vi "timming_array_to_digital_waveform.vi"(3 "timing array":dbl[](array[numeric])) -> (0 "digital waveform":digitalwaveform(waveform)={"t0"=timestamp(0 s since 1904-01-01), "dt"=0.0, "Y"={"transitions"=[], "data"=[]}, "error"={"status"=FALSE, "code"=37421928, "source"=""}})   [LabVIEW 2011]
doc: "takes the timing info recieved from the DG645 Delay generator and transforms it into a digital waveform graph.\nMakes sure, all timings are setup in reference to t0!"
uses:
  <vilib>/Waveform/DWDTOps.llb/DWDT Boolean Array to Digital.vi
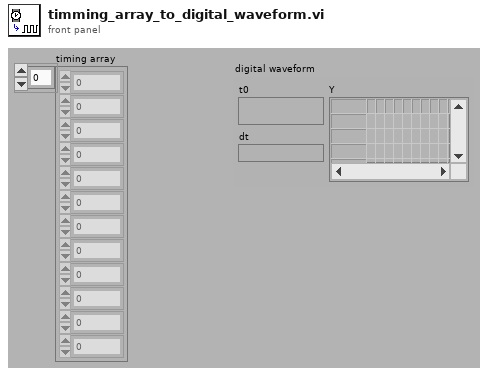
[diagram p1: front panel]
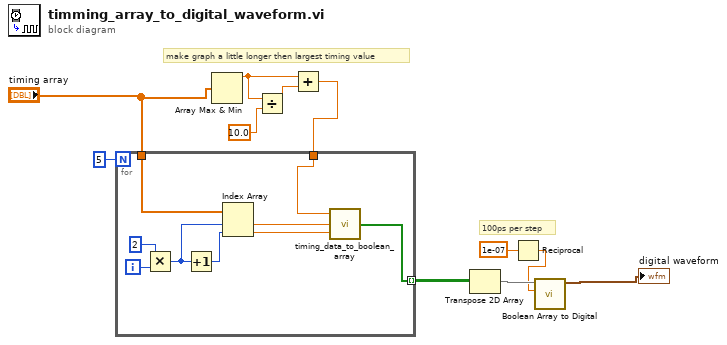
[diagram p0: block diagram]
diagram:
  # "100ps per step"
  # "make graph a little longer then largest timing value"
  n1 = Array Max & Min(array="timing array") -> (max value=w5:dbl)  [unwired: 3 out]
  n2 = Divide(x=w5, y=10.0) -> (x/y=w4:dbl)
  n3 = Add(x=w5, y=w4) -> (x+y=w3:dbl)
  n4 = for {
    N: 5 -> [_]
    tunnel: [w18] -> w10 mode=indexing
    tunnel: w3 -> [w17]
    tunnel: "timing array" -> [w16]
    i -> [w20]
    n5 = Multiply(x=2, y=w20) -> (x*y=w12:i32)
    n6 = Increment(x=w12) -> (x+1=w15:i32)
    n7 = Index Array(array=w16, index #1=w12, index #2=w15) -> (element #1=w14:dbl, element #2=w13:dbl)
    n8 = call "timing_data_to_boolean_array.vi"("end time [us]"=w13, "start time [us]"=w14, "overall length [us]"=w17) -> ("boolean timing array"=w18:bool[])  [unwired: 1 in]
  }
  n9 = Transpose 2D Array(2D array=w10) -> (transposed array=w9:bool[][])
  n10 = Reciprocal(x=1e-07) -> (1/x=w1:dbl)
  n11 = call-poly <vilib>:"Boolean Array to Digital.vi"("sample rate"=w1, "boolean array"=w9) -> ("digital waveform"=→"digital waveform":digitalwaveform)  [unwired: 8 in, 1 out]
